vi "BRig_dataExp_guiState_DAB.vi"() -> (2 "output_guiState_DAB":i32)   [LabVIEW 2014]
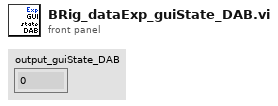
[diagram p1: front panel]
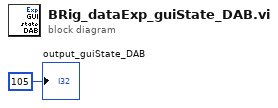
[diagram p0: block diagram]
diagram:
  "output_guiState_DAB" <- 105 ("output_iBlock")
